vi "setindex.vi"(6 "Index":i32, 8 "error in":errorcluster, 9 "Phase (rad)":dbl, 10 "Amplitude (V)":dbl, 11 "Resonance Curve Data in":refnum<class "Resonance Curve Data.lvclass">) -> (0 "error out":errorcluster, 3 "Resonance Curve Data out":refnum<class "Resonance Curve Data.lvclass">)   [LabVIEW 2020, in "Resonance Curve Data.lvclass"]
uses:
  Resonance Curve Data.lvclass
  Resonance Curve Data.lvclass/Resonance Curve Data.ctl
panel:
  # "Given a pair of amplitude and phase measurements, in-place update the resonance curve data at the specified index"
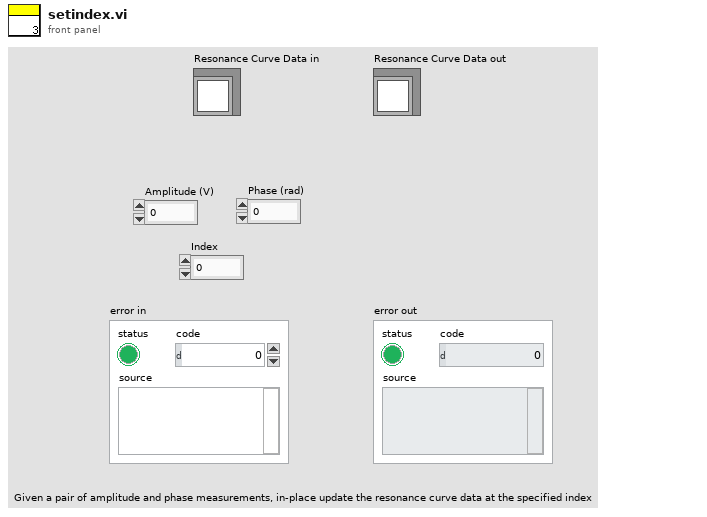
[diagram p1: front panel]
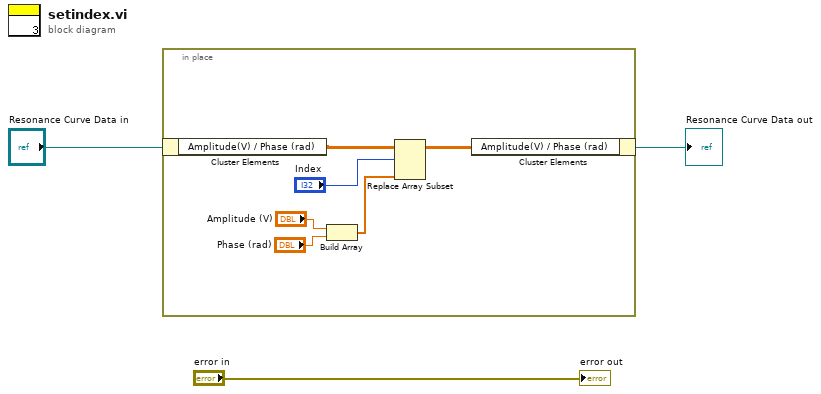
[diagram p0: block diagram]
diagram:
  n1 = in-place {
    n2 = in-place-cluster #1("Resonance Curve Data in") -> ("Amplitude(V) / Phase (rad)"=w9:dbl[][])
    n3 = Build Array("Amplitude (V)", "Phase (rad)") -> (w5:dbl[])
    n4 = Replace Array Subset(array=w9, new element=w5, index (row)="Index") -> (w4:dbl[][])  [unwired: 1 in]
    n5 = in-place-cluster #1("Amplitude(V) / Phase (rad)"=w4) -> (→"Resonance Curve Data out":refnum<class "Resonance Curve Data.lvclass">)
  }
  "error out" <- "error in"
